vi "Overview Mouse Move.vi"(8 "error in":errorcluster, 10 "Coords":T1, 11 "XYGraphOverview in":refnum<class "XYGraphOverview.lvclass">) -> (0 "error out":errorcluster, 3 "XYGraphOverview out":refnum<class "XYGraphOverview.lvclass">)   [LabVIEW 2020, in "XYGraphOverview.lvlib" / "XYGraphOverview.lvclass"]
uses:
  XYGraphOverview.lvclass
  <vilib>/Utility/miscctls.llb/LVPoint32TypeDef.ctl
  XYGraphOverview.lvclass/XYGraphOverview.ctl
  Read Highlight Block Color.vi
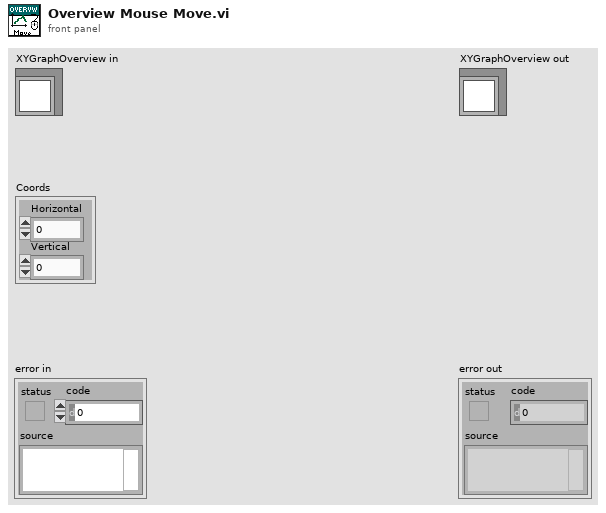
[diagram p1: front panel]
types:
  T1 = typedef "LVPoint32TypeDef.ctl" = cluster{"Horizontal":i32, "Vertical":i32}
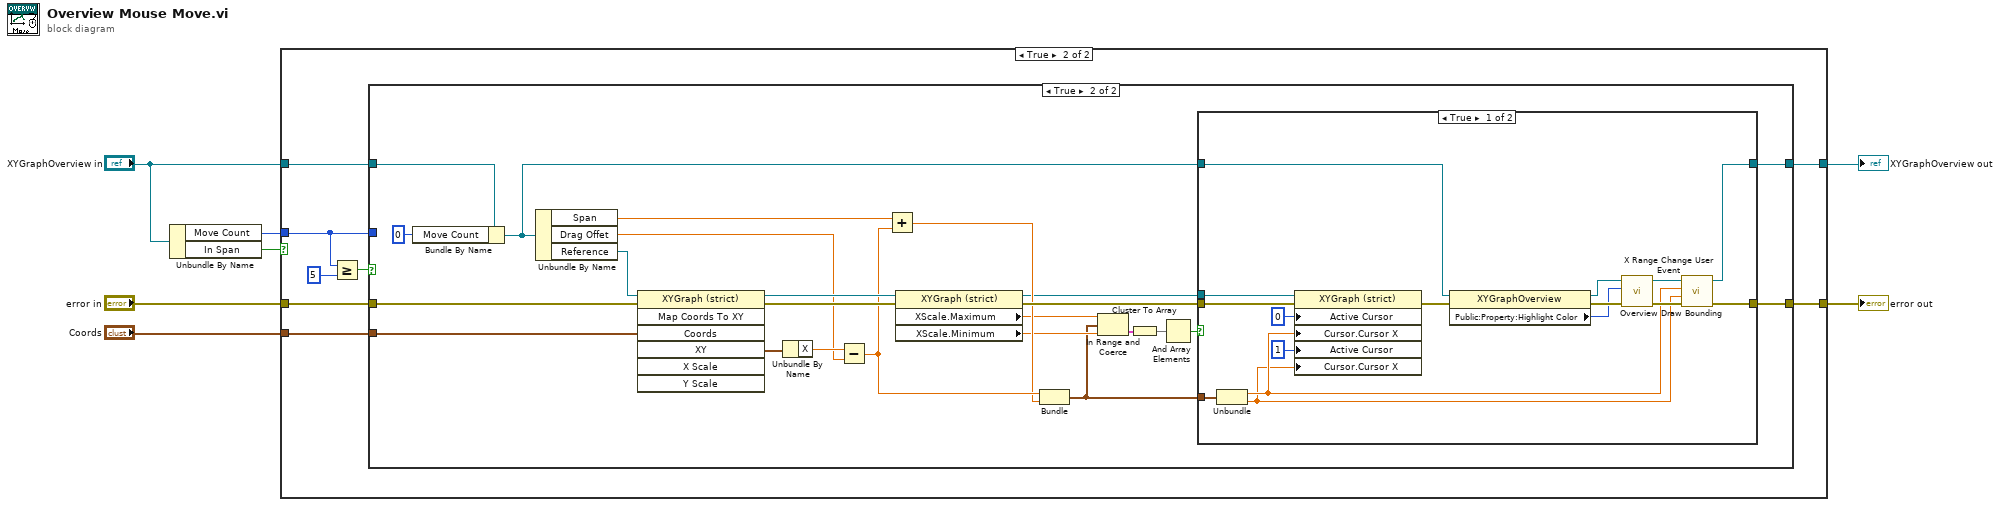
[diagram p0: block diagram]
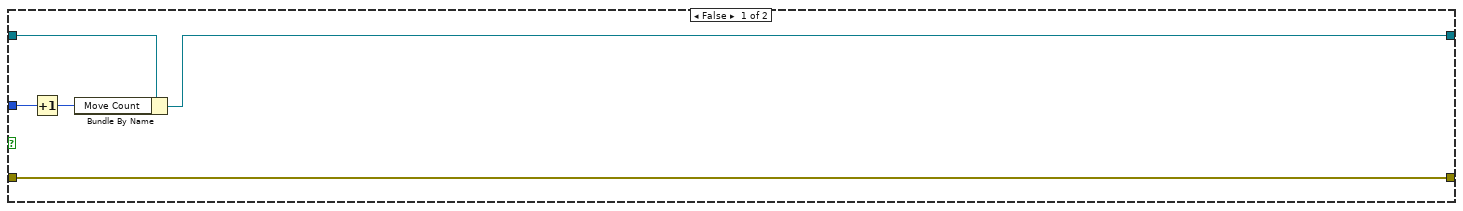
[diagram p3: hidden frame]
diagram:
  n1 = Unbundle By Name("XYGraphOverview in") -> ("Move Count"=w2:u32, "In Span"=w1:bool)
  n2 = case shown="True" w1 {
    tunnel: "Coords" -> [_ w17]
    tunnel: [w8 w16] -> w7
    tunnel: [w9 w15] -> w6
    tunnel: "error in" -> [w8 w14]
    tunnel: "XYGraphOverview in" -> [w9 w13]
    tunnel: w2 -> [_ w11]
    frame False {
    }
    frame True {
      n3 = Greater Or Equal?(x=w11, y=u32 5) -> (x >= y?=w10:bool)
      n4 = case shown="True" w10 {
        tunnel: w17 -> [_ w46]
        tunnel: [w22 w45] -> w16
        tunnel: [w18 w44] -> w15
        tunnel: w13 -> [w21 w25]
        tunnel: w14 -> [w22 w37]
        tunnel: w11 -> [w20 _]
        frame False {
          n5 = Increment(x=w20) -> (x+1=w19:u32)
          n6 = Bundle By Name(cluster=w21, "Move Count"=w19) -> (w18:refnum<class "XYGraphOverview.lvclass">)
        }
        frame True {
          n7 = Bundle By Name(cluster=w25, "Move Count"=u32 0) -> (w24:refnum<class "XYGraphOverview.lvclass">)
          n8 = Unbundle By Name(w24) -> ("Span"=w35:dbl, "Drag Offet"=w36:dbl, "Reference"=w38:refnum<vi>)
          n9 = invoke on="Invoke Node" class="XYGraph (strict)" method="Map Coords To XY"(reference=w38, error in=w37, "Coords"=w46) -> (reference out=w39:refnum<vi>, error out=w41:errorcluster, "XY"=w43:cluster{"X":dbl, "Y":dbl})  [unwired: 4 in, 4 out]
          n10 = Unbundle By Name(w43) -> ("X"=w42:dbl)
          n11 = Subtract(x=w42, y=w36) -> (x-y=w34:dbl)
          n12 = Add(x=w35, y=w34) -> (x+y=w33:dbl)
          n13 = property on="Property Node" class="XYGraph (strict)"(reference=w39, error in=w41) -> (reference out=w27:refnum<vi>, error out=w40:errorcluster, "XScale.Maximum"=w32:dbl, "XScale.Minimum"=w31:dbl)
          n14 = Bundle(w34, w33) -> (w26:cluster{dbl, dbl})  [unwired: 1 in]
          n15 = In Range and Coerce(upper limit=w32, x=w26, lower limit=w31) -> (In Range?=w30:cluster{bool, bool})  [unwired: 1 out]
          n16 = Cluster To Array(cluster=w30) -> (array=w29:bool[])
          n17 = And Array Elements(Boolean array=w29) -> (logical AND=w28:bool)
          n18 = case shown="True" w28 {
            tunnel: w40 -> [w60 w63]
            tunnel: w24 -> [w50 w64]
            tunnel: [w54 w63] -> w45
            tunnel: [w55 w64] -> w44
            tunnel: w27 -> [w59 _]
            tunnel: w26 -> [w58 _]
            frame True {
              n19 = Unbundle(w58) -> (w53:dbl, w52:dbl)
              n20 = property class="XYGraph (strict)"(reference=w59, error in=w60, "Active Cursor"=u32 0, "Cursor.Cursor X"=w53, "Active Cursor"=u32 1, "Cursor.Cursor X"=w52) -> (error out=w51:errorcluster)  [unwired: 1 out]
              n21 = property class="XYGraphOverview"(reference=w50, error in=w51) -> (reference out=w48:refnum<class "XYGraphOverview.lvclass">, error out=w49:errorcluster, "Public:Property:Highlight Color"=w47:u32)
              n22 = call "Overview Draw Bounding.vi"("error in (no error)"=w49, "Color"=w47, "XYGraphOverview in"=w48) -> ("error out"=w57:errorcluster, "XYGraphOverview out"=w56:refnum<class "XYGraphOverview.lvclass">)  [unwired: 7 in]
              n23 = call "X Range Change User Event.vi"("error in (no error)"=w57, "Upper Range"=w52, "Lower Range"=w53, "XYGraphOverview in"=w56) -> ("error out"=w54:errorcluster, "XYGraphOverview out"=w55:refnum<class "XYGraphOverview.lvclass">)  [unwired: 6 in]
            }
            frame False {
            }
          }
        }
      }
    }
  }
  "error out" <- w7
  "XYGraphOverview out" <- w6
